vi "Write HumTECs.vi"(8 "error in (no error)":errorcluster, 10 "HumTECs":T1={"tecSP"="Filter In", "tecEn"="Filter In"}, 11 "cPAS in":refnum<class "cPAS.lvclass">) -> (0 "error out":errorcluster, 3 "cPAS out":refnum<class "cPAS.lvclass">)   [LabVIEW 2015, in "cPAS.lvclass"]
uses:
  cPAS.lvclass
  cPAS.lvclass/cPAS.ctl
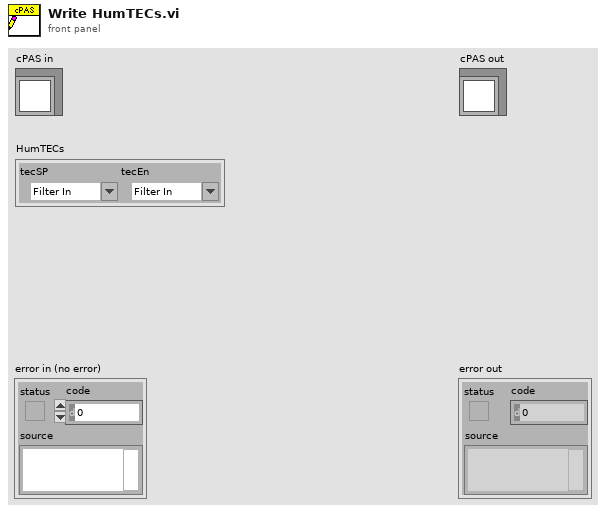
[diagram p1: front panel]
types:
  T1 = cluster{"tecSP":refnum<k21>, "tecEn":refnum<k21>}
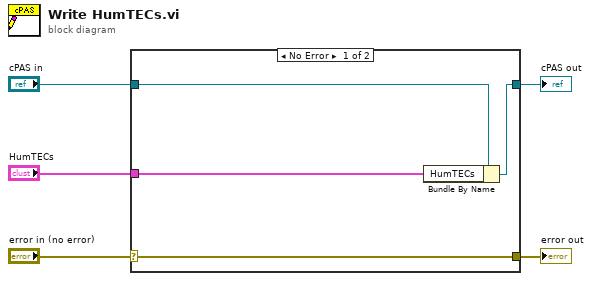
[diagram p0: block diagram]
diagram:
  n1 = case shown="No Error" "error in (no error)" {
    selector: "error in (no error)" -> [w9 w10]
    tunnel: [w9 w10] -> w4
    tunnel: [w7 w11] -> w2
    tunnel: "cPAS in" -> [w8 w11]
    tunnel: "HumTECs" -> [w6 _]
    frame No Error {
      n2 = Bundle By Name(cluster=w8, "HumTECs"=w6) -> (w7:refnum<class "cPAS.lvclass">)
    }
    frame Error {
    }
  }
  "error out" <- w4
  "cPAS out" <- w2
